vi "Angle Distance VI.vi"(9 "current angle":dbl(knob) scale=-180.0..180.0, 11 "target angle":dbl(knob) scale=-180.0..180.0) -> (2 "distance":dbl)   [LabVIEW 2020]
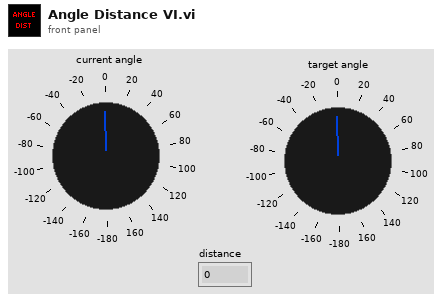
[diagram p1: front panel]
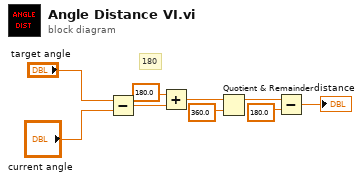
[diagram p0: block diagram]
diagram:
  # "180"
  n1 = Subtract(x="target angle", y="current angle") -> (x-y=w7:dbl)
  n2 = Add(x=180.0, y=w7) -> (x+y=w5:dbl)
  n3 = Quotient & Remainder(x=w5, y=360.0) -> (x-y*floor(x/y)=w3:dbl)  [unwired: 1 out]
  n4 = Subtract(x=w3, y=180.0) -> (x-y=→"distance":dbl)
